vi "Open Array of SVs.vi"(8 "error in (no error)":errorcluster, 9 "SV Name":string, 10 "SV":refnum<k21>[](array[refnum]), 11 "AEgIS Shared Variables in":refnum<class "Circus Shared Variables.lvclass">[](array[class])) -> (0 "error out":errorcluster, 3 "AEgIS Shared Variables out":refnum<class "Circus Shared Variables.lvclass">[](array[class]))   [LabVIEW 2026, in "TALOS.lvlib" / "Classes.lvlib" / "Circus Shared Variables.lvclass"]
doc: "Use this VI to open a connection to multiple Shared Variables. If the array of Var Ref is given in input, or the array of AEgIS SVs, the list is used and all the connections are opened; otherwise, the VI looks on the network for all the SVs with a name matching with the one given in input, and then tries to open a connection with all the SVs found."
uses:
  Circus Shared Variables.lvclass
  Ancestor/Ancestor/Ancestor.lvclass/Ancestor.ctl
  Circus Shared Variables.lvclass/Circus Shared Variables.ctl
  FGV/Error Memory/Get Error Description.vi
  Support VIs/Get PC name.vi
  Ancestor/Ancestor/Read ID.vi
  Support VIs/Get Class Name.vi
  <vilib>/Utility/error.llb/Clear Errors.vi
  FGV/Error Memory/Error Memory Core.vi
  <vilib>/AdvancedString/Delimited String to 1D String Array.vi
  <vilib>/AdvancedString/Delimited String to 1D String Array (string).vi
  Support VIs/Circus Root Path.vi
  FGV/Error Memory/Error Crt Lvl checker.vi
  FGV/Error Memory/Error Memory Core.vi/40c8088d-b597-4017-91af-faa98e00292e.vi
  FGV/Error Memory/Error Memory Core.vi/d4a3ab98-063c-4e44-b43d-fbdcfe6c2be2.vi
  Support VIs/Global Memory.vi
  <vilib>/Utility/LVClass/Get LV Class Name.vi
  Support VIs/Is in Packed Library.vi
  Support VIs/TALOS Root path.vi
  Support VIs/Read CSV worksheet.vi
  Support VIs/Global Constants.vi
  <vilib>/Utility/error.llb/General Error Handler.vi
  <vilib>/Utility/config.llb/Open Config Data.vi
  <vilib>/Utility/config.llb/Get Section Names.vi
  <vilib>/Utility/config.llb/Get Key Names.vi
  <vilib>/Utility/config.llb/Read Key.vi
  <vilib>/Utility/config.llb/Read Key (String).vi
  <vilib>/Utility/config.llb/Close Config Data.vi
  Support VIs/Error Log.vi
  Ancestor/Ancestor/Ancestor.lvclass
  <vilib>/Comparison/Equal/Equal Functor/Equal Functor.lvclass
  <resource>/objmgr/ni.var.rc
  TALOS.lvlib
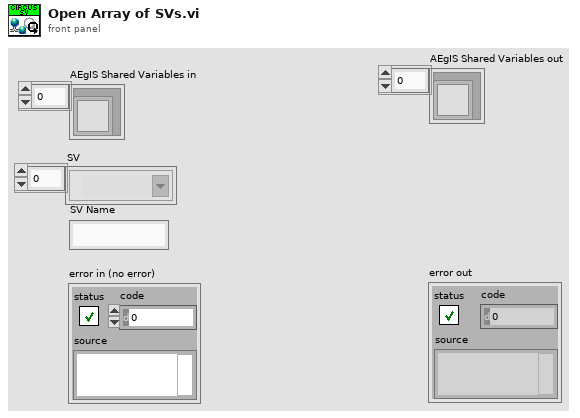
[diagram p1: front panel]
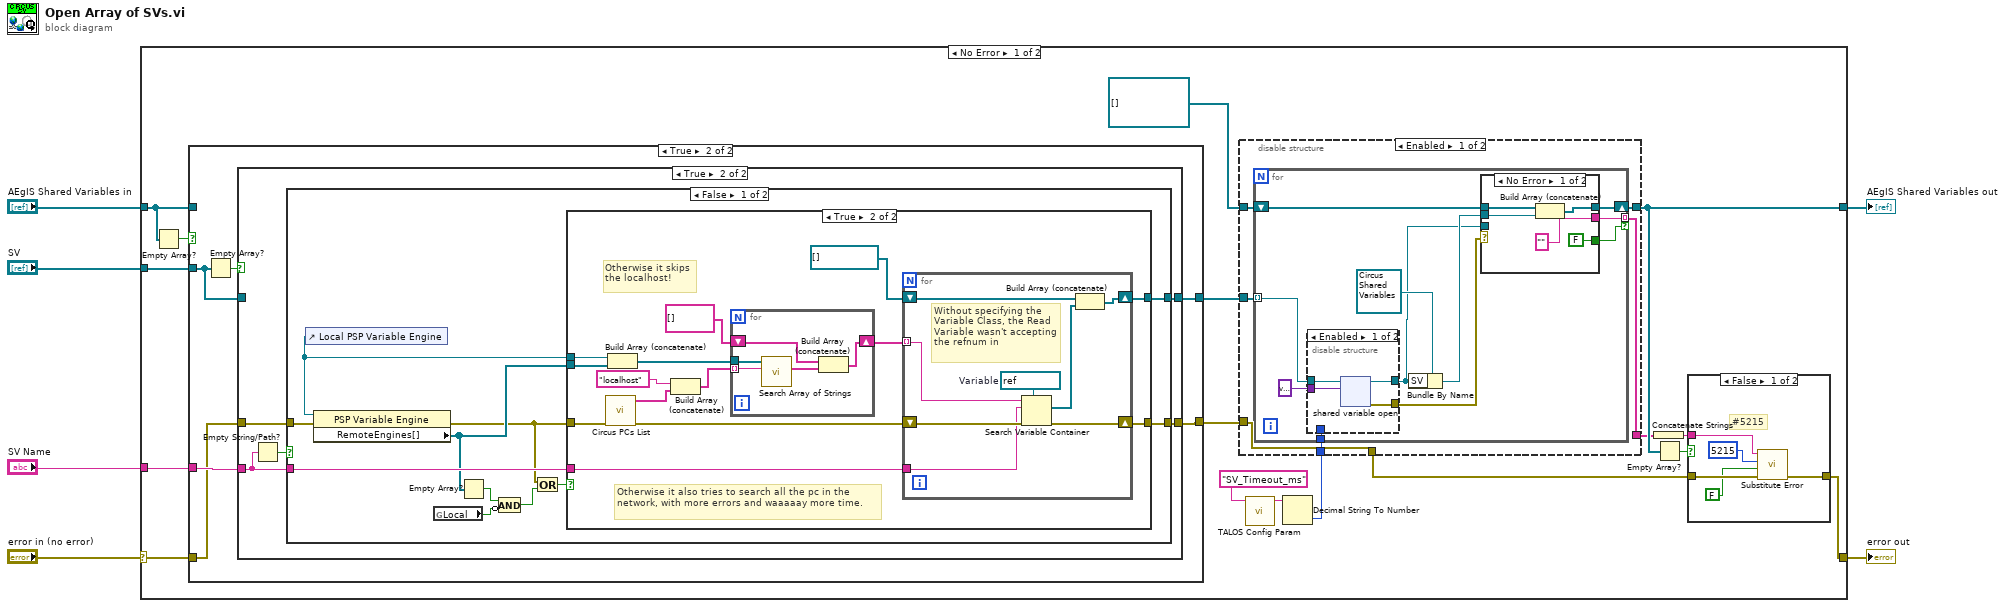
[diagram p0: block diagram]
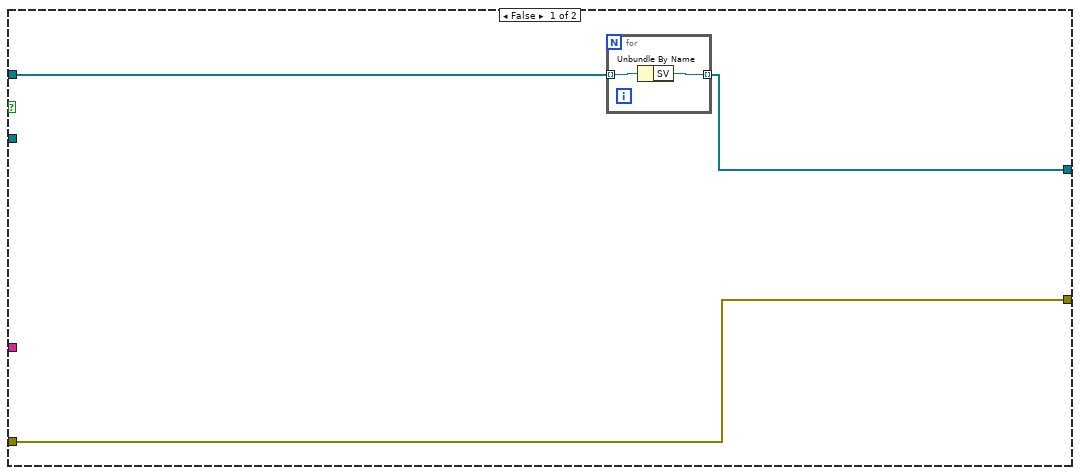
[diagram p2: hidden frame]
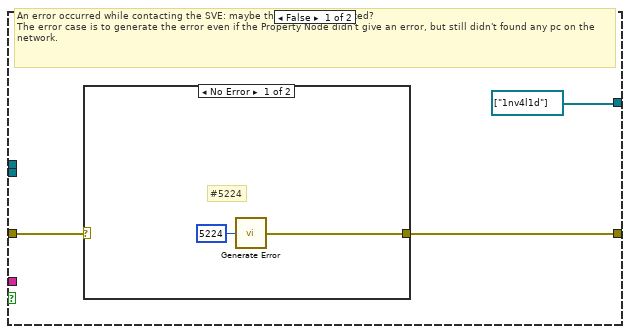
[diagram p4: hidden frame]
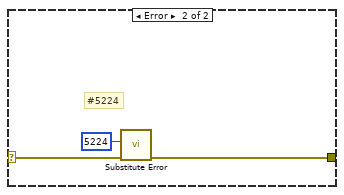
[diagram p5: hidden frame]
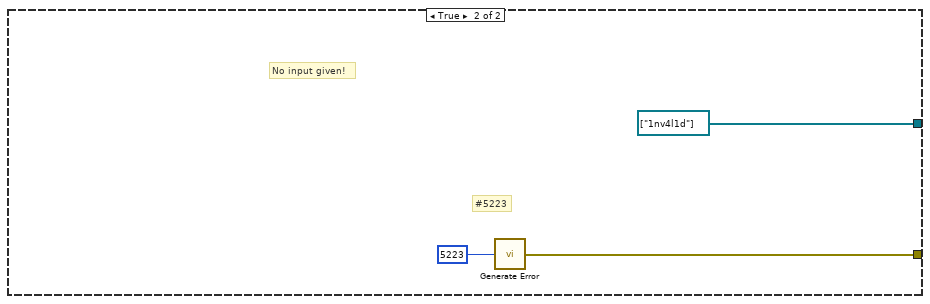
[diagram p6: hidden frame]
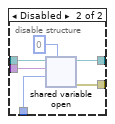
[diagram p7: hidden frame]
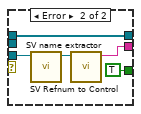
[diagram p8: hidden frame]
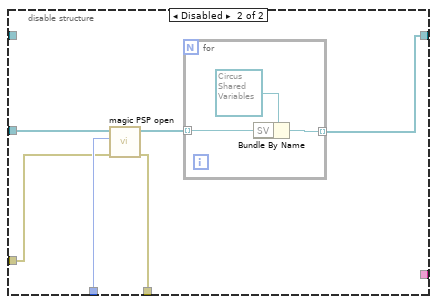
[diagram p9: hidden frame]
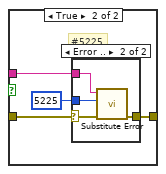
[diagram p10: hidden frame]
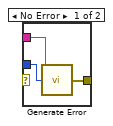
[diagram p11: hidden frame]
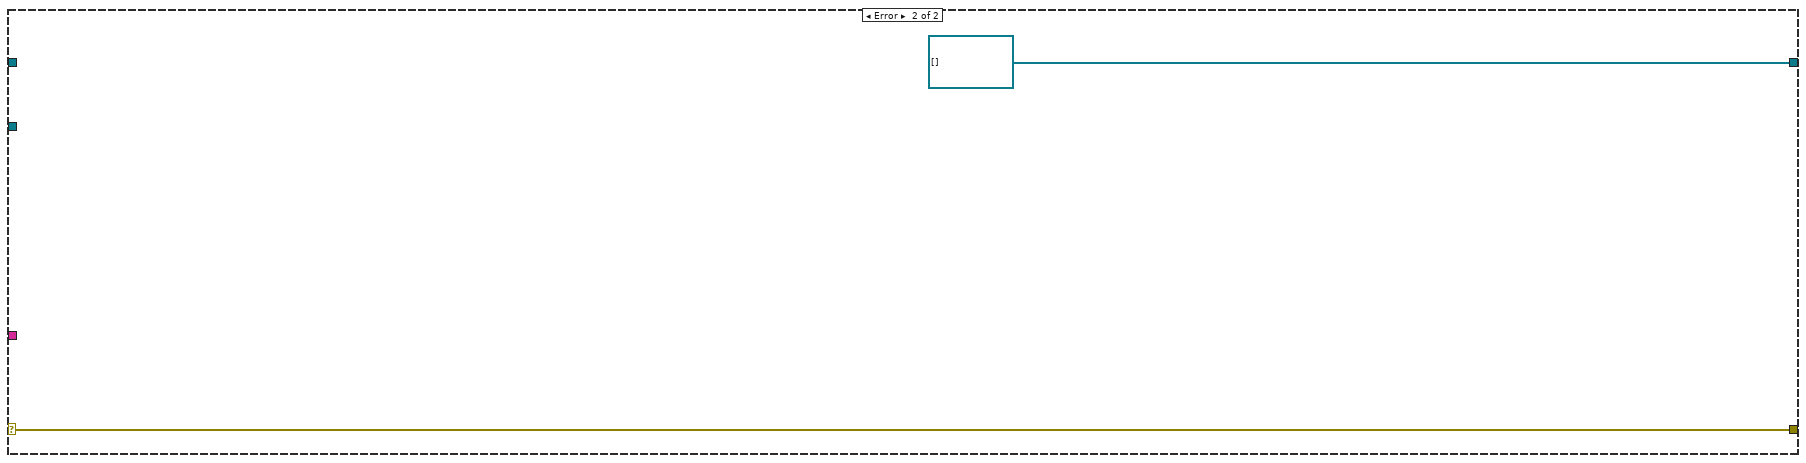
[diagram p12: hidden frame]
diagram:
  n1 = case shown="No Error" "error in (no error)" {
    selector: "error in (no error)" -> [w21 w154]
    tunnel: [w9 w154] -> w5
    tunnel: "SV" -> [w23 _]
    tunnel: "SV Name" -> [w22 _]
    tunnel: [w15 refnum<class "Circus Shared Variables.lvclass">[] [] ("AEgIS Shared Variables out")] -> w2
    tunnel: "AEgIS Shared Variables in" -> [w19 _]
    frame No Error {
      n2 = Empty Array?(array=w19) -> (empty?=w20:bool)
      n3 = case shown="True" w20 {
        tunnel: w23 -> [_ w34]
        tunnel: w22 -> [_ w33]
        tunnel: w21 -> [w24 w32]
        tunnel: w19 -> [w26 _]
        tunnel: [w24 w30] -> w11
        tunnel: [w25 w29] -> w17
        frame False {
          n4 = for {
            tunnel: w26 -> [w28] mode=indexing
            tunnel: [w27] -> w25 mode=indexing
            n5 = Unbundle By Name(w28) -> ("SV"=w27:refnum<k21>)
          }
        }
        frame True {
          n6 = Empty Array?(array=w34) -> (empty?=w31:bool)
          n7 = case shown="True" w31 {
            tunnel: w32 -> [w36 w41]
            tunnel: w33 -> [_ w38]
            tunnel: w34 -> [w35 _]
            tunnel: [w36 w40] -> w30
            tunnel: [w35 w39] -> w29
            frame False {
            }
            frame True {
              n8 = Empty String/Path?(string/path=w38) -> (empty?=w37:bool)
              n9 = case shown="False" w37 {
                tunnel: w41 -> [w51 _]
                tunnel: w38 -> [w50 _]
                tunnel: [w49 w90] -> w40
                tunnel: [w48 refnum<k21>[] ["1nv4l1d"]] -> w39
                frame False {
                  n10 = control-ref of="Local PSP Variable Engine"() -> (w52:refnum<k21>)
                  n11 = property class="PSP Variable Engine"(reference=w52, error in=w51) -> (error out=w43:errorcluster, "RemoteEngines[]"=w44:refnum<k21>[])  [unwired: 1 out]
                  n12 = global read "Global Constants.vi" "Local"() -> (w45:bool)
                  n13 = Empty Array?(array=w44) -> (empty?=w46:bool)
                  n14 = Compound Arithmetic op=AND(w46, invert w45) -> (w47:bool)
                  n15 = Or(x=w43, y=w47) -> (x .or. y?=w42:bool)
                  n16 = case shown="True" w42 {
                    tunnel: w52 -> [_ w72]
                    tunnel: w43 -> [w55 w70]
                    tunnel: w50 -> [_ w68]
                    tunnel: w44 -> [_ w67]
                    tunnel: [w54 w66] -> w49
                    tunnel: [refnum<k21>[] ["1nv4l1d"] w65] -> w48
                    frame False {
                      # "An error occurred while contacting the SVE: maybe the firewall is blocked?\nThe error case is to generate the error even if the Property Node didn't give an error, but still didn't found any pc on the network."
                      n17 = case shown="No Error" w55 {
                        selector: w55 -> [_ w60]
                        tunnel: [w57 w58] -> w54
                        frame No Error {
                          # "#5224"
                          n18 = call "Generate Error.vi"("Error Code"=5224) -> ("error out"=w57:errorcluster)  [unwired: 6 in]
                        }
                        frame Error {
                          # "#5224"
                          n19 = call "Substitute Error.vi"("error in (no error)"=w60, "Error Code"=5224) -> ("error out"=w58:errorcluster)  [unwired: 9 in]
                        }
                      }
                    }
                    frame True {
                      # "Otherwise it also tries to search all the pc in the network, with more errors and waaaaay more time."
                      # "Otherwise it skips the localhost!"
                      n20 = call "Circus PCs List.vi"("error in (no error)"=w70) -> ("error out"=w69:errorcluster, "PC List out"=w63:string[])  [unwired: 9 in]
                      n21 = Build Array (concatenate)(w72, w67) -> (w74:refnum<k21>[])
                      n22 = Build Array (concatenate)("localhost", w63) -> (w62:string[])
                      n23 = for {
                        tunnel: w74 -> [w87]
                        tunnel: w62 -> [w84] mode=indexing
                        shift-right: [w86] -> w73
                        shift-left: string[] [] -> [w83]
                        n24 = call "Search Array of Strings.vi"("search string"=w84, "Search array"=w87) -> ("found elements"=w85:string[])  [unwired: 8 in, 1 out]
                        n25 = Build Array (concatenate)(w83, w85) -> (w86:string[])
                      }
                      n26 = for {
                        shift-right: [w81] -> w66
                        shift-left: w69 -> [w80]
                        tunnel: w73 -> [w79] mode=indexing
                        shift-right: [w76] -> w65
                        shift-left: refnum<k21>[] [] -> [w78]
                        tunnel: w68 -> [w75]
                        w82 = refnum<k21> refnum  # Variable
                        # "Without specifying the Variable Class, the Read Variable wasn't accepting the refnum in"
                        n27 = Search Variable Container(7:w82, 8:w80, 10:w75, 11:w79) -> (0:w81:errorcluster, 2:w77:refnum<k21>[])  [unwired: 2 in, 1 out]
                        n28 = Build Array (concatenate)(w78, w77) -> (w76:refnum<k21>[])
                      }
                    }
                  }
                }
                frame True {
                  # "#5223"
                  # "No input given!"
                  n29 = call "Generate Error.vi"("Error Code"=5223) -> ("error out"=w90:errorcluster)  [unwired: 6 in]
                }
              }
            }
          }
        }
      }
      n30 = call "TALOS Config Param.vi"("Parameter Name"="SV_Timeout_ms") -> ("Output"=w14:string)  [unwired: 9 in, 1 out]
      n31 = Decimal String To Number(string=w14) -> (number=w13:i32)  [unwired: 2 in, 1 out]
      n32 = disable-structure shown="Enabled" {
        disable-tunnel: refnum<class "Circus Shared Variables.lvclass">[] [] ("AEgIS Shared Variables out") -> [w96 _]
        disable-tunnel: w17 -> [w95 w133]
        disable-tunnel: [w94 w130] -> w15
        disable-tunnel: w13 -> [w93 w132]
        disable-tunnel: w11 -> [w92 w129]
        disable-tunnel: [w92 w128] -> w10
        disable-tunnel: [w91 _] -> w8
        frame Enabled {
          n33 = for {
            shift-right: [w103] -> w94
            shift-left: w96 -> [w105]
            tunnel: w95 -> [w102] mode=indexing
            tunnel: w93 -> [w100]
            tunnel: [w98] -> w91 mode=indexing if=w97
            n34 = disable-structure shown="Enabled" {
              disable-tunnel: variant ("data type") -> [w111 w116]
              disable-tunnel: [w110 w115] -> w99
              disable-tunnel: w102 -> [w109 w117]
              disable-tunnel: [w108 w114] -> w101
              disable-tunnel: w100 -> [_ w112]
              frame Enabled {
                n35 = shared-variable-open(w109, w111) -> (w110:refnum<k21>, w108:errorcluster)  [unwired: 1 in]
              }
              frame Disabled {
                n36 = shared-variable-open(w117, w116, w112, u32 0 ("buffer size in elements")) -> (w115:refnum<k21>, w114:errorcluster)  [unwired: 1 in]
              }
            }
            n37 = Bundle By Name(cluster=refnum<class "Circus Shared Variables.lvclass"> refnum ("AEgIS Shared Variables in"), "SV"=w99) -> (w104:refnum<class "Circus Shared Variables.lvclass">)
            n38 = case shown="No Error" w101 {
              tunnel: w105 -> [w122 w127]
              tunnel: w104 -> [w121 _]
              tunnel: [w120 w127] -> w103
              tunnel: w99 -> [_ w126]
              tunnel: ["" ("String") w124] -> w98
              tunnel: [FALSE TRUE] -> w97
              frame No Error {
                n39 = Build Array (concatenate)(w122, w121) -> (w120:refnum<class "Circus Shared Variables.lvclass">[])
              }
              frame Error {
                n40 = call "SV Refnum to Control.vi"("shared variable refnum in"=w126) -> ("Shared Variable Control Out"=w125:refnum<k21>)  [unwired: 9 in, 1 out]
                n41 = call "SV name extractor.vi"("Refnum in"=w125) -> ("String"=w124:string)  [unwired: 10 in]
              }
            }
          }
        }
        frame Disabled {
          n42 = call "magic PSP open.vi"("error in (no error)"=w129, "timeout (ms)"=w132, "vars in"=w133) -> ("error out"=w128:errorcluster, "Vars out"=w131:refnum<k21>[])  [unwired: 6 in, 1 out]
          n43 = for {
            tunnel: w131 -> [w135] mode=indexing
            tunnel: [w134] -> w130 mode=indexing
            n44 = Bundle By Name(cluster=refnum<class "Circus Shared Variables.lvclass"> refnum ("AEgIS Shared Variables in"), "SV"=w135) -> (w134:refnum<class "Circus Shared Variables.lvclass">)
          }
        }
      }
      n45 = Concatenate Strings(w8) -> (w7:string)
      n46 = Empty Array?(array=w15) -> (empty?=w16:bool)
      n47 = case shown="False" w16 {
        tunnel: [w140 w145] -> w9
        tunnel: w10 -> [w141 w143]
        tunnel: w7 -> [w137 w142]
        frame False {
          # "#5215"
          n48 = call "Substitute Error.vi"("error in (no error)"=w141, "Error/Warning"=FALSE, "Error Code"=5215, "Optional String"=w137) -> ("error out"=w140:errorcluster)  [unwired: 7 in]
        }
        frame True {
          # "#5225"
          n49 = case shown="Error .." w143 {
            selector: w143 -> [_ w152]
            tunnel: [w148 w151] -> w145
            tunnel: 5225 ("Error Code") -> [w147 w150]
            tunnel: w142 -> [w146 w149]
            frame No Error {
              n50 = call "Generate Error.vi"("Optional String"=w146, "Error Code"=w147) -> ("error out"=w148:errorcluster)  [unwired: 5 in]
            }
            frame Error {
              n51 = call "Substitute Error.vi"("error in (no error)"=w152, "Error Code"=w150, "Optional String"=w149) -> ("error out"=w151:errorcluster)  [unwired: 8 in]
            }
          }
        }
      }
    }
    frame Error {
    }
  }
  "error out" <- w5
  "AEgIS Shared Variables out" <- w2
